vi "InitSP.vi"(8 "error in (no error)":errorcluster, 11 "SimulationParameter in":refnum<class "SimulationParameter.lvclass">) -> (0 "error out":errorcluster, 3 "SimulationParameter out":refnum<class "SimulationParameter.lvclass">)   [LabVIEW 2017, in "SimulationParameter.lvclass"]
uses:
  SimulationParameter.lvclass
  SimulationParameter.lvclass/SimulationParameter.ctl
  <vilib>/drjdpowell/SQLite Library/SQL Connection/Execute SQL (Single Integer).vi
  <vilib>/drjdpowell/SQLite Library/SQLite.lvlib
  <vilib>/drjdpowell/SQLite Library/SQL Connection/Connection.lvclass
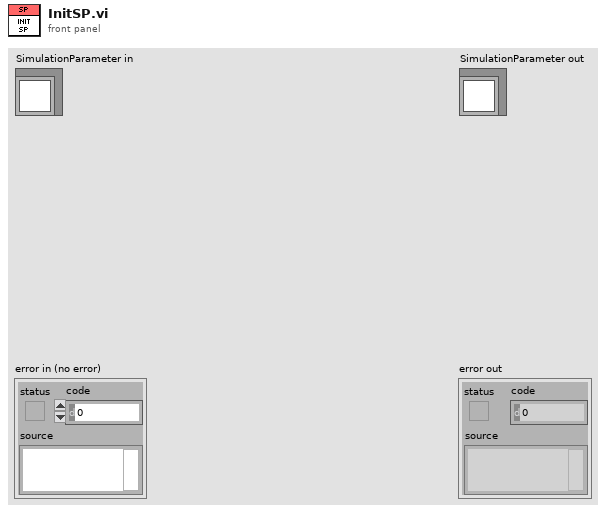
[diagram p1: front panel]
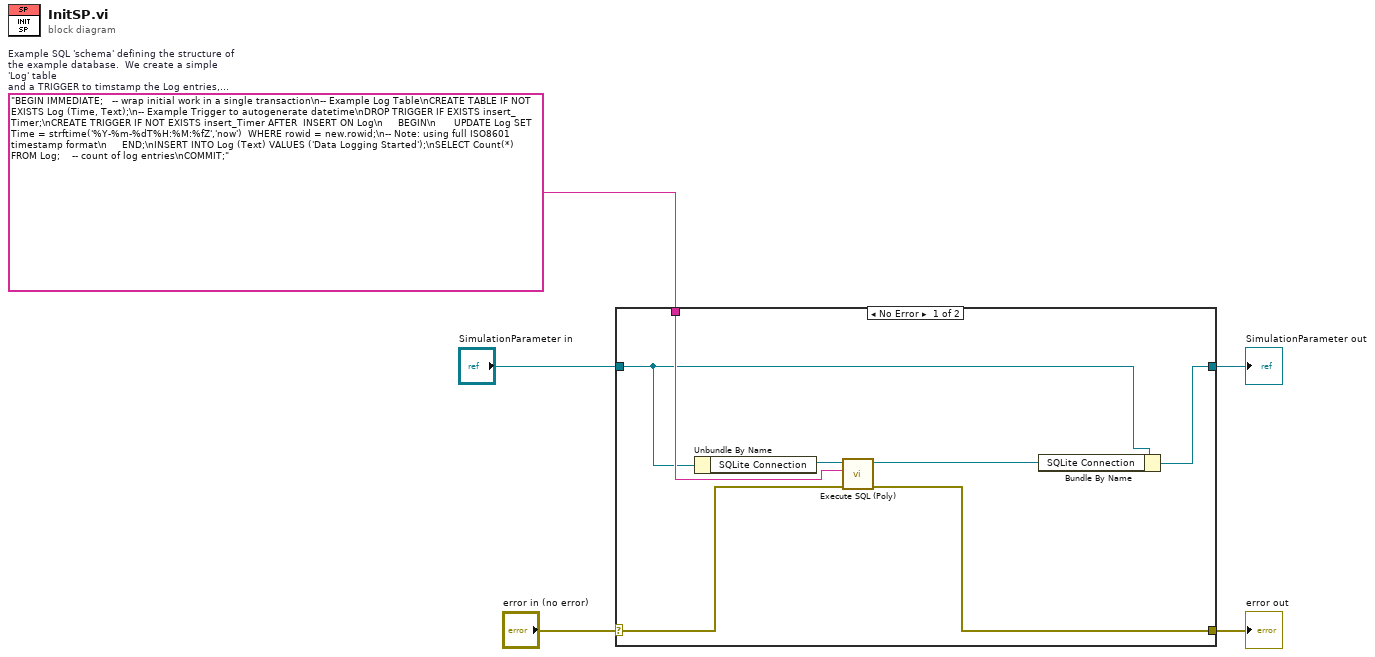
[diagram p0: block diagram]
diagram:
  w1 = "BEGIN IMMEDIATE;   -- wrap initial work in a single transaction\n-- Example Log Table\nCREATE TABLE IF NOT EXISTS Log (Time, Text);\n-- Example Trigger to autogenerate datetime\nDROP TRIGGER IF EXISTS insert_Timer;\nCREATE TRIGGER IF NOT EXISTS insert_Timer AFTER  INSERT ON Log\n     BEGIN\n      UPDATE Log SET Time = strftime('%Y-%m-%dT%H:%M:%fZ','now')  WHERE rowid = new.rowid;\n-- Note: using full ISO8601 timestamp format\n     END;\nINSERT INTO Log (Text) VALUES ('Data Logging Started');\nSELECT Count(*) FROM Log;    -- count of log entries\nCOMMIT;"  # Example SQL 'schema' defining the structure of the example database.  We create a simple 'Log' table and a TRIGGER to timstamp the Log entries, then a simple 'Data' table
  n1 = case shown="No Error" "error in (no error)" {
    selector: "error in (no error)" -> [w7 w14]
    tunnel: [w6 w14] -> w4
    tunnel: [w8 w13] -> w2
    tunnel: "SimulationParameter in" -> [w9 w13]
    tunnel: w1 -> [w10 _]
    frame No Error {
      n2 = Unbundle By Name(w9) -> ("SQLite Connection"=w11:refnum<class "Connection.lvclass">)
      n3 = call-poly <vilib>:"Execute SQL (Poly).vi"("error in (no error)"=w7, "SQL"=w10, "SQLite Connection in"=w11) -> ("error out"=w6:errorcluster, "SQLite Connection out"=w12:refnum<class "Connection.lvclass">)  [unwired: 6 in, 1 out]
      n4 = Bundle By Name(cluster=w9, "SQLite Connection"=w12) -> (w8:refnum<class "SimulationParameter.lvclass">)
    }
    frame Error {
    }
  }
  "error out" <- w4
  "SimulationParameter out" <- w2
